vi "Send Reset Min-Max.vi"(7 "Message Priority (Normal)":T1=enum."Normal", 8 "error in (no error)":errorcluster, 10 "Reset Min/Max (T: Reset)":bool=TRUE, 11 "Message Enqueuer":refnum<class "Message Enqueuer.lvclass">) -> (0 "error out":errorcluster, 3 "Message Enqueuer out":refnum<class "Message Enqueuer.lvclass">)   [LabVIEW 2016, in "LS218.lvlib" / "Reset Min-Max Msg.lvclass"]
doc: "Sends the <B>LS218.lvlib:Reset Min-Max Msg.lvclass</B> message.\n\n<B>LS218.lvlib:LS218.lvclass:Reset Min-Max.vi</B> Description:\n\nThis VI resets the minimum and maximum data for all inputs."
uses:
  Reset Min-Max Msg.lvclass
  <vilib>/ActorFramework/Message Enqueuer/Message Enqueuer.lvclass
  <vilib>/ActorFramework/Message Enqueuer/Message Priority.ctl
  C:/Program Files (x86)/National Instruments/LabVIEW 2016/vi.lib/ActorFramework/Message/Message.lvclass
  Reset Min-Max Msg.lvclass/Reset Min-Max Msg.ctl
  <vilib>/ActorFramework/Message Enqueuer/Message Enqueuer.lvclass/Message Enqueuer.ctl
  <vilib>/ActorFramework/Message Priority Queue/Priority Enqueue.vi
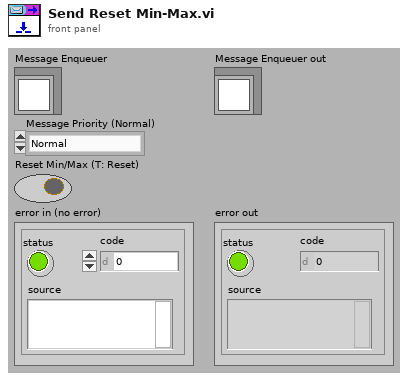
[diagram p1: front panel]
types:
  T1 = typedef "Actor Framework.lvlib/Message Enqueuer.lvclass/Message Priority.ctl" = enum16{"Low", "Normal", "High"}
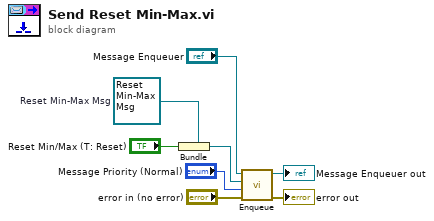
[diagram p0: block diagram]
diagram:
  w2 = refnum<class "Reset Min-Max Msg.lvclass"> refnum  # Reset Min-Max Msg
  n1 = Bundle(cluster=w2, "Reset Min/Max (T: Reset)") -> (w5:refnum<class "Reset Min-Max Msg.lvclass">)
  n2 = call <vilib>:"Enqueue.vi"("error in (no error)"="error in (no error)", "Message Priority (Normal)"="Message Priority (Normal)", "Message"=w5, "Message Enqueuer in"="Message Enqueuer") -> ("error out"=→"error out":errorcluster, "Message Enqueuer out"=→"Message Enqueuer out":refnum<class "Message Enqueuer.lvclass">)  [unwired: 6 in]
